vi "array gen 1.vi"(7 "Points":i32, 10 "End":dbl, 11 "Start":dbl) -> (3 "Array":dbl[](array[numeric]))   [LabVIEW 2023]
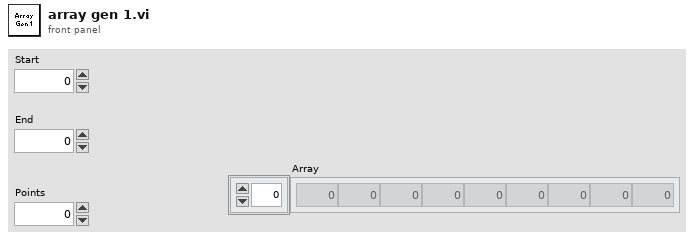
[diagram p1: front panel]
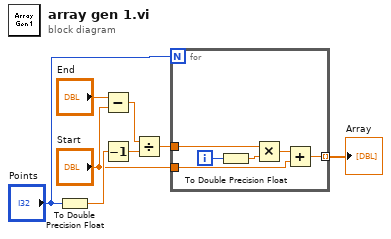
[diagram p0: block diagram]
diagram:
  n1 = To Double Precision Float(number="Points") -> (double precision float=w6:dbl)
  n2 = Subtract(x="End", y="Start") -> (x-y=w7:dbl)
  n3 = Decrement(x=w6) -> (x-1=w5:dbl)
  n4 = Divide(x=w7, y=w5) -> (x/y=w3:dbl)
  n5 = for {
    N: "Points" -> [_]
    tunnel: w3 -> [w13]
    tunnel: "Start" -> [w10]
    tunnel: [w9] -> w1 mode=indexing
    i -> [w14]
    n6 = To Double Precision Float(number=w14) -> (double precision float=w12:dbl)
    n7 = Multiply(x=w13, y=w12) -> (x*y=w11:dbl)
    n8 = Add(x=w11, y=w10) -> (x+y=w9:dbl)
  }
  "Array" <- w1
